vi "get_gpib_data.vi"(8 "error in (no error)":errorcluster, 11 "GPIB Rsrc":string[](array[string])) -> (0 "error out":errorcluster, 1 "GPIB I/F name":string[](array[string]), 2 "Primary Address":u16[](array[numeric]), 3 "GPIB Inst ID":string[](array[string]))   [LabVIEW 2015]
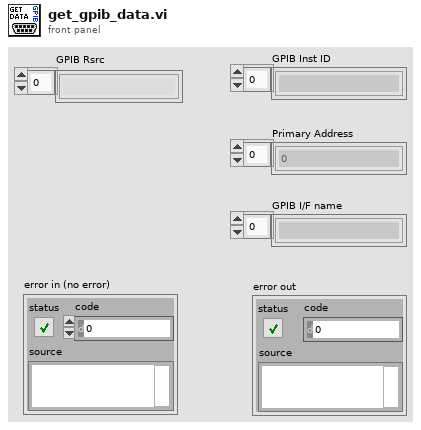
[diagram p1: front panel]
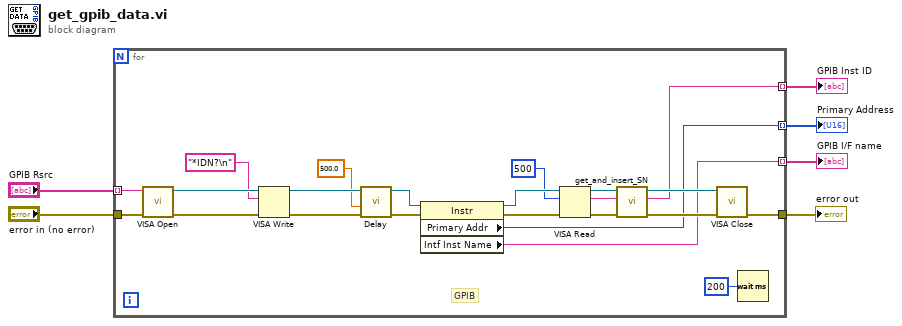
[diagram p0: block diagram]
diagram:
  n1 = for {
    tunnel: [w18] -> w3 mode=indexing
    tunnel: [w26] -> w4
    tunnel: [w10] -> w5 mode=indexing
    tunnel: [w21] -> w6 mode=indexing
    tunnel: "error in (no error)" -> [w17]
    tunnel: "GPIB Rsrc" -> [w16] mode=indexing
    # "GPIB"
    n2 = call "VISA Open.vi"("error in (no error)"=w17, "VISA resource name"=w16) -> ("error out"=w24:errorcluster, "VISA resource name out"=w25:refnum<visa-resource-name>)  [unwired: 8 in]
    n3 = VISA Write(VISA resource name=w25, write buffer="*IDN?\n", error in (no error)=w24) -> (VISA resource name out=w15:refnum<visa-resource-name>, error out=w19:errorcluster)  [unwired: 1 out]
    n4 = call "Delay.vi"("error in (no error)"=w19, "milliseconds to wait"=500.0) -> ("error out"=w20:errorcluster)  [unwired: 9 in]
    n5 = property class="Instr"(reference=w15, error in=w20) -> (reference out=w22:refnum<visa-resource-name>, error out=w23:errorcluster, "Primary Addr"=w21:u16, "Intf Inst Name"=w18:string)
    n6 = VISA Read(VISA resource name=w22, byte count=u32 500, error in (no error)=w23) -> (VISA resource name out=w12:refnum<visa-resource-name>, read buffer=w11:string, error out=w13:errorcluster)  [unwired: 1 out]
    n7 = call "get_and_insert_SN.vi"("error in (no error)"=w13, "read buffer in"=w11, "VISA Refnum in"=w12) -> ("error out"=w27:errorcluster, "read buffer out"=w10:string, "VISA Refnum out"=w28:refnum<visa-resource-name>)  [unwired: 6 in]
    n8 = call "VISA Close.vi"("error in (no error)"=w27, "VISA resource name"=w28) -> ("error out"=w26:errorcluster)  [unwired: 9 in]
    n9 = Wait (ms)(milliseconds to wait=u32 200) -> ()  [unwired: 1 out]
  }
  "Primary Address" <- w6
  "GPIB Inst ID" <- w5
  "error out" <- w4
  "GPIB I/F name" <- w3
